vi "Write Port.vi"(0 "Simulada in":refnum<class "Simulada.lvclass">, 5 "VISA resource name":refnum<visa-resource-name>, 9 "Port":u16, 11 "error in (no error)":errorcluster, 12 "Set Port":bool[](array[boolean])) -> (4 "Simulada out":refnum<class "Simulada.lvclass">, 6 "VISA resource name out":refnum<visa-resource-name>, 15 "error out":errorcluster)   [LabVIEW 2020, in "Simulada.lvclass"]
uses:
  Simulada.lvclass
  Abstract/Serial Device/Serial Device.lvclass
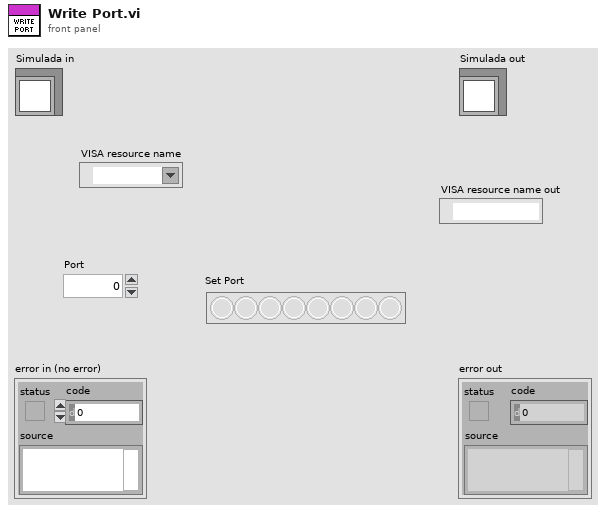
[diagram p1: front panel]
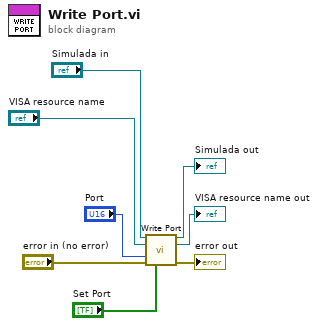
[diagram p0: block diagram]
diagram:
  n1 = call-parent "Write Port.vi"("Serial Device in"="Simulada in", "VISA resource name"="VISA resource name", "Port"="Port", "error in (no error)"="error in (no error)", "Set Port"="Set Port") -> ("Serial Device out"=→"Simulada out":refnum<class "Simulada.lvclass">, "VISA resource name out"=→"VISA resource name out":refnum<visa-resource-name>, "error out"=→"error out":errorcluster)  [unwired: 8 in]
